vi "FIFO Read.vi"(0 "FPGA Ref":T3, 5 "Elements Available":T2, 11 "error in":errorcluster, 12 "Imaging Protocol":T1) -> (4 "FPGA VI Reference Out":T3, 6 "Data arrays cluster":T4, 10 "Elements Remaining (Ch0)":u32, 14 "Image Time Elements Remaining":u32, 15 "error out":errorcluster)   [LabVIEW 2020]
uses:
  Typedefs/Data arrays cluster.ctl
  RIG-SPECIFIC FILES/FPGA Refs/FPGA Ref.ctl
  Acquisition/Typedefs/FIFO elements available.ctl
  Typedefs/Imaging Protocols enum.ctl
  <vilib>/Utility/error.llb/Error Cluster From Error Code.vi
  <vilib>/rvi/errors/niLvFpgaAdjustHostInterfaceError.vi
  <vilib>/rvi/interface/nirviReadWriteControl/nirviReadWriteControl.xnode
  <vilib>/rvi/interface/nirviMethod/nirviMethod.xnode
  <vilib>/rvi/errors/niLvFpgaMergeErrorWithErrorCode.vi
  <vilib>/FPGAPlugInAG/Dynamic/niLvFpga_ReadFifo_Dynamic.vi
  NiFpgaLv.dll
  <vilib>/rvi/interface/Simulation/niFpgaSimulationCallBeginRW.vi
panel:
  out "x pixels count":u16[](array[numeric])
  out "y count array":u16[](array[numeric])
  out "x pixels current":u16
  out "y count":u16
  out "Continuous Time Elements Remaining":u32
  out "Ref time Elements Remaining":u32
  out "Elements Remaining (Ch1)":u32
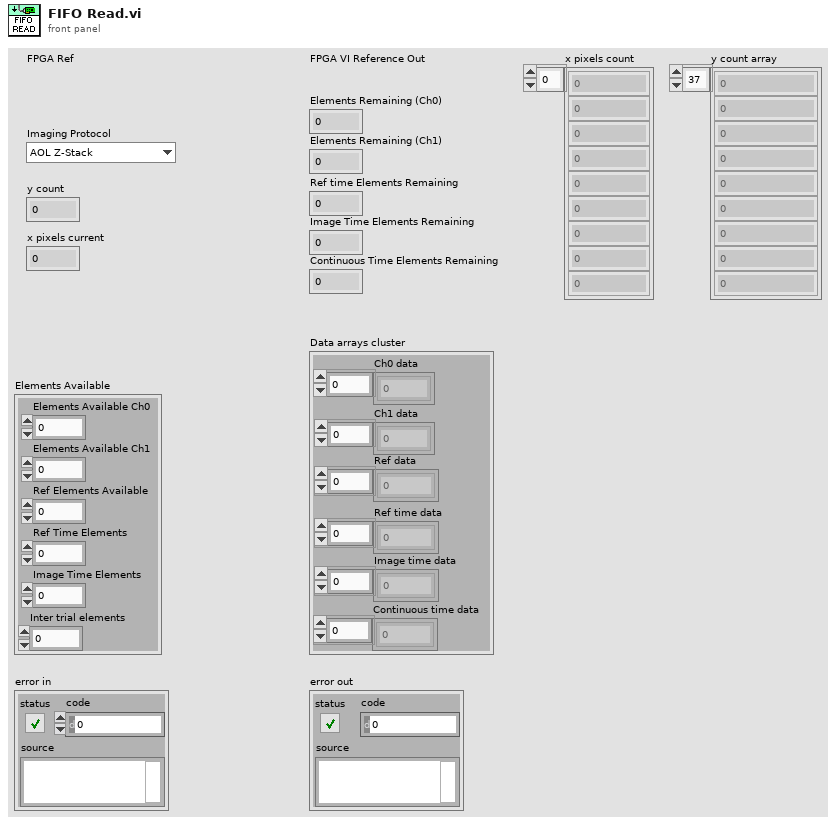
[diagram p1: front panel]
types:
  T1 = typedef "Imaging Protocols enum.ctl" = enum16{"AOL Z-Stack", "Motor Z Stack", "Functional Acquisition", "Single Plane Acquisition", "Volume Acquisition", "Live Imaging", "Live Plane Imaging", "Live Volume Imaging"}
  T2 = typedef "FIFO elements available.ctl" = cluster{"Elements Available Ch0":u32, "Elements Available Ch1":u32, "Ref Elements Available":u32, "Ref Time Elements":u32, "Image Time Elements":u32, "Inter trial elements":u32}
  T3 = typedef "FPGA Ref.ctl" = refnum<k20>
  T4 = typedef "Data arrays cluster.ctl" = cluster{"Ch0 data":u32[], "Ch1 data":u32[], "Ref data":u32[], "Ref time data":u64[], "Image time data":u64[], "Continuous time data":u64[]}
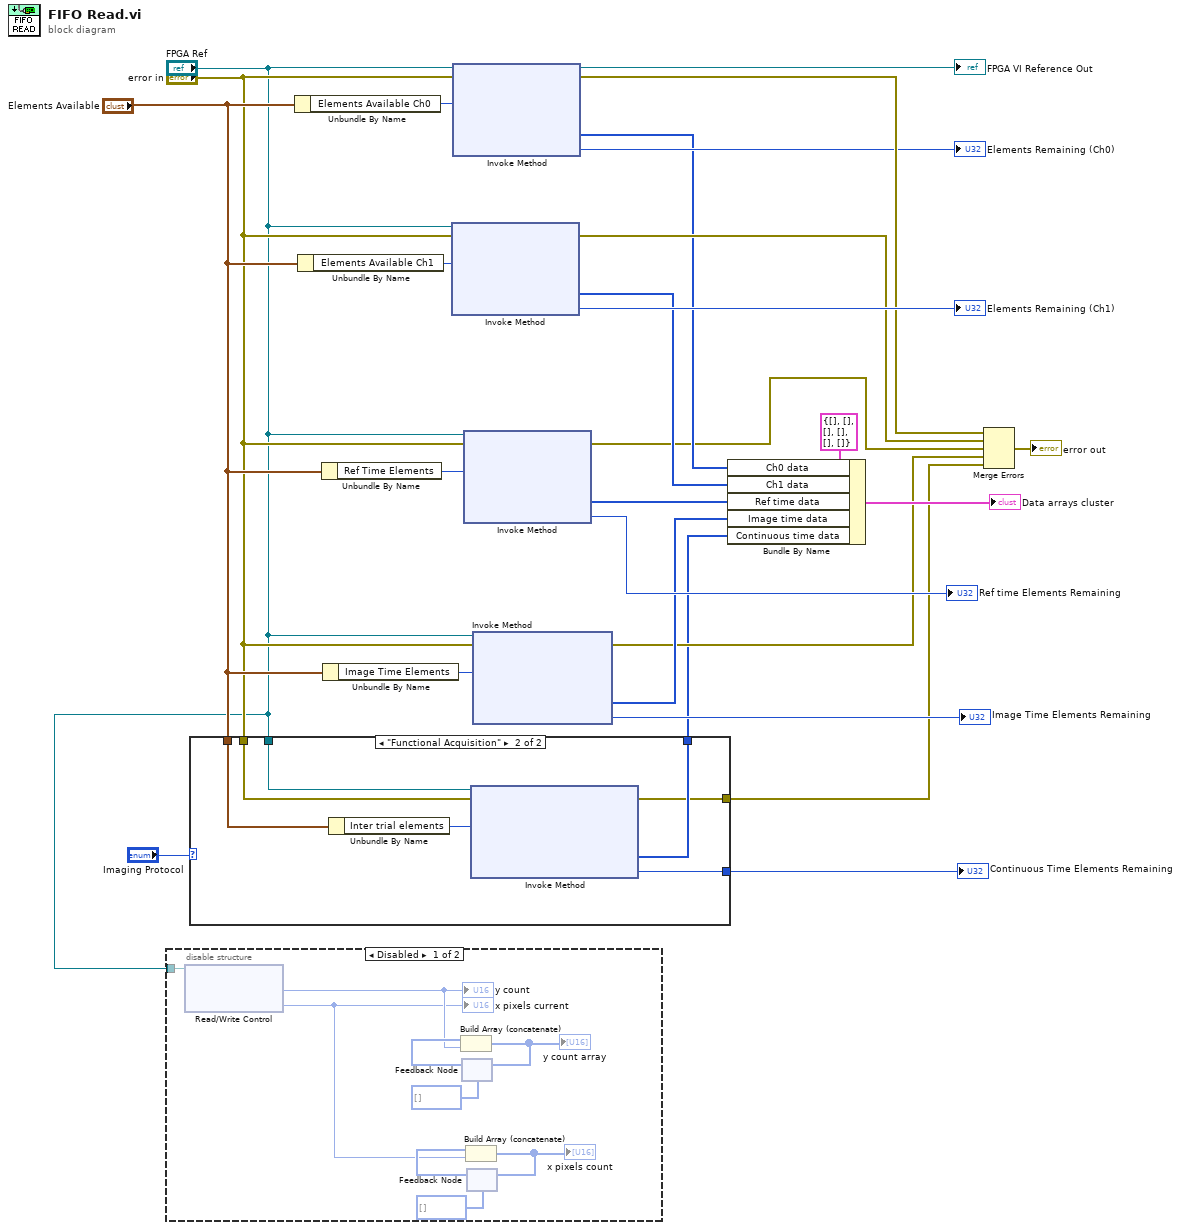
[diagram p0: block diagram]
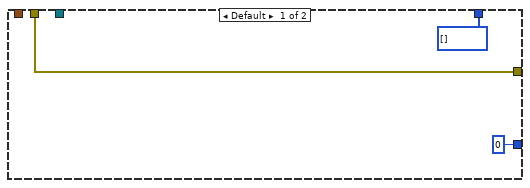
[diagram p3: hidden frame]
diagram:
  n1 = disable-structure shown="Disabled" {
    disable-tunnel: "FPGA Ref" -> [w36 _]
    frame Disabled {
      n2 = xnode "Read/Write Control"("FPGA VI Reference In"=w36) -> ("y count"=w33:u16, "x pixels current"=w28:u16)  [unwired: 1 in, 2 out]
      "y count" <- w33
      "x pixels current" <- w28
      n3 = feedback #1(u16[] []) -> (w34:u16[])
      n4 = Build Array (concatenate)(w34, w33) -> (w32:u16[])
      "y count array" <- w32
      n5 = feedback-in #1(w32) -> ()
      n6 = feedback #2(u16[] []) -> (w30:u16[])
      n7 = Build Array (concatenate)(w30, w28) -> (w31:u16[])
      "x pixels count" <- w31
      n8 = feedback-in #2(w31) -> ()
    }
    frame Enabled {
    }
  }
  n9 = case shown="\"Functional Acquisition\"" "Imaging Protocol" {
    tunnel: "Elements Available" -> [_ w45]
    tunnel: "FPGA Ref" -> [_ w44]
    tunnel: [u64[] [] ("Data") w43] -> w6
    tunnel: [u32 0 ("Elements Remaining") w42] -> w5
    tunnel: [w39 w40] -> w3
    tunnel: "error in" -> [w39 w41]
    frame Default {
    }
    frame "Functional Acquisition" {
      n10 = Unbundle By Name(w45) -> ("Inter trial elements"=w46:u32)
      n11 = xnode ("Invoke Method")("FPGA VI Reference In"=w44, "error in"=w41, "Number of Elements"=w46) -> ("error out"=w40:errorcluster, "Data"=w43:u64[], "Elements Remaining"=w42:u32)  [unwired: 1 in, 1 out]
    }
  }
  "Continuous Time Elements Remaining" <- w5
  n12 = Unbundle By Name("Elements Available") -> ("Elements Available Ch0"=w17:u32)
  n13 = Unbundle By Name("Elements Available") -> ("Elements Available Ch1"=w16:u32)
  n14 = Unbundle By Name("Elements Available") -> ("Ref Time Elements"=w15:u32)
  n15 = Unbundle By Name("Elements Available") -> ("Image Time Elements"=w12:u32)
  n16 = xnode ("Invoke Method")("FPGA VI Reference In"="FPGA Ref", "error in"="error in", "Number of Elements"=w16) -> ("error out"=w23:errorcluster, "Data"=w19:u32[], "Elements Remaining"=→"Elements Remaining (Ch1)":u32)  [unwired: 1 in, 1 out]
  n17 = xnode ("Invoke Method")("FPGA VI Reference In"="FPGA Ref", "error in"="error in", "Number of Elements"=w17) -> ("FPGA VI Reference Out"=→"FPGA VI Reference Out":T3, "error out"=w24:errorcluster, "Data"=w20:u32[], "Elements Remaining"=→"Elements Remaining (Ch0)":u32)  [unwired: 1 in]
  n18 = xnode ("Invoke Method")("FPGA VI Reference In"="FPGA Ref", "error in"="error in", "Number of Elements"=w15) -> ("error out"=w9:errorcluster, "Data"=w13:u64[], "Elements Remaining"=→"Ref time Elements Remaining":u32)  [unwired: 1 in, 1 out]
  n19 = xnode ("Invoke Method")("FPGA VI Reference In"="FPGA Ref", "error in"="error in", "Number of Elements"=w12) -> ("error out"=w8:errorcluster, "Data"=w10:u64[], "Elements Remaining"=→"Image Time Elements Remaining":u32)  [unwired: 1 in, 1 out]
  n20 = Bundle By Name(cluster=T4 {"Ch0 data"=[], "Ch1 data"=[], "Ref data"=[], "Ref time data"=[], "Image time data"=[], "Continuous time data"=[]} ("Data arrays cluster"), "Ch0 data"=w20, "Ch1 data"=w19, "Ref time data"=w13, "Image time data"=w10, "Continuous time data"=w6) -> (→"Data arrays cluster":T4)
  n21 = Merge Errors(w24, w23, w9, w8, w3) -> (→"error out":errorcluster)
